vi "Teleop.vi"(10 "Match Info":T1={"Autonomous Elapsed Seconds"=0.0, "TeleOp Elapsed Seconds"=0.0, "Disabled Elapsed Seconds"=0.0, "Visited Autonomous"=FALSE, "Visited TeleOp"=FALSE, "Visited Disabled"=FALSE, "Autonomous Settings"={"Autonomous Style"=enum."Independent", "VI Refnum"=refnum}}, 11 "Call Context":T2) -> ()   [LabVIEW 2016]
doc: "This VI is called for each TeleOp packet received from the DS where the robot is not disabled. It is often used to read from the joysticks and update I/O or to update setpoints for timed control loops. It should complete and return within 20 milliseconds or it may miss DS packets."
uses:
  <vilib>/Rock Robotics/WPI/DriverStation/WPI_DriverStationDerivedRobotMode.ctl
  <vilib>/Rock Robotics/WPI/DriverStation/WPI_DriverStationMatch Info.ctl
  <vilib>/Rock Robotics/WPI/ThirdParty/CanMotor/TalonSRX/WPI_CANTalonSRX_APIFeedbackSelect.ctl
  <vilib>/Rock Robotics/WPI/ThirdParty/CanMotor/TalonSRX/WPI_CANTalonSRX_APIControlMode.ctl
  <vilib>/Rock Robotics/WPI/Utilities/WPI_GetSetVariantRefNum.vi
  <vilib>/Rock Robotics/Network Tables/NT Write Boolean Array.vi
  <vilib>/Rock Robotics/Network Tables/NT Write Numeric Array.vi
  <vilib>/Rock Robotics/Network Tables/NT Read Boolean.vi
  <vilib>/Rock Robotics/Network Tables/NT Read Number.vi
  Robot Global Data.vi
panel:
  out "Battery Voltage":dbl
  out "Current":dbl
  out "SensorPosRotations":dbl
  out "Motor output Plot":cluster{"Applied Throttle":dbl}(graph)
  out "Target RPM":dbl
  out "SensorRPM Velocity RPM":dbl
  out "Applied Output":dbl
  out "Speed Closed Loop Plots":cluster{dbl, "Sensor Velocity":dbl}(graph)
  in  "Enable":bool=TRUE
  in  "Reset":bool
  out "Table":string[][](table)
  out "Encoder Velocity":dbl
  out "Sample Slider 0":dbl(slide) scale=0.0..5.0
  out "Sample Boolean 1":bool
  out "Sample Boolean 0":bool
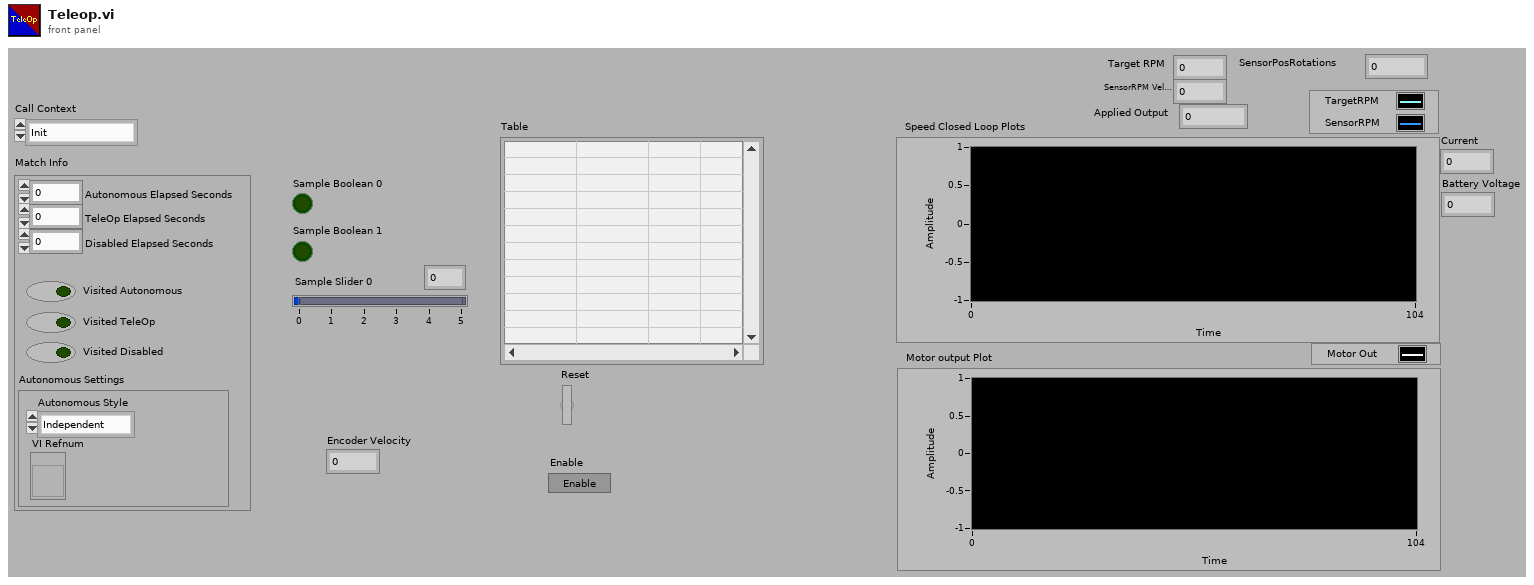
[diagram p1: front panel]
types:
  T1 = typedef "WPI_DriverStationMatch Info.ctl" = cluster{"Autonomous Elapsed Seconds":dbl, "TeleOp Elapsed Seconds":dbl, "Disabled Elapsed Seconds":dbl, "Visited Autonomous":bool, "Visited TeleOp":bool, "Visited Disabled":bool, "Autonomous Settings":cluster{"Autonomous Style":enum16{"Iterative", "Independent"}, "VI Refnum":refnum<vi>}}
  T2 = typedef "WPI_DriverStationDerivedRobotMode.ctl" = enum16{"Init", "Execute", "Stop"}
  T3 = typedef "WPI_CANTalonSRX_APIFeedbackSelect.ctl" = enum16{"Digital Quadrature Encoder", "Analog Potentiometer", "Analog Encoder", "Count on Quad-A (Rising-Edge)", "Count on Quad-A (Falling-Edge)", "CTR Magnetic Enc (Absolute)", "CTR Magnetic Enc (Relative)", "Pulse Width"}
  T4 = typedef "WPI_JoystickDevRef.ctl" = cluster{"Device":T5}
  T5 = typedef "WPI_JoystickDeviceEnum.ctl" = enum16{"USB 0", "USB 1", "USB 2", "USB 3", "USB 4", "USB 5"}
  T6 = typedef "WPI_MotorControlDeviceRef.ctl" = cluster{"DeviceStatus":errorcluster, "Type":T7, "PWM":cluster{"PWM Channel":T8, "DeadBand":T9}, "CAN":cluster{"Device Number":u8, "SetOutput VI Ref":variant, "GetOutput VI Ref":variant, "Enable VI Ref":variant, "Disable VI Ref":variant, "Data":variant}, "Invert":bool}
  T7 = typedef "WPI_MotorControlType.ctl" = enum16{"PWM", "CAN"}
  T8 = typedef "FPGA_DIOPWMChannel.ctl" = enum8{"PWM 0", "PWM 1", "PWM 2", "PWM 3", "PWM 4", "PWM 5", "PWM 6", "PWM 7", "PWM 8", "PWM 9", "PWM MXP 0", "PWM MXP 1", "PWM MXP 2", "PWM MXP 3", "PWM MXP 4", "PWM MXP 5", "PWM MXP 6", "PWM MXP 7", "PWM MXP 8", "PWM MXP 9", "Invalid"}
  T9 = typedef "WPI_PWMDeadband.ctl" = cluster{"Name":string, "maxPositivePwm":i32, "minPositivePwm":i32, "centerPwm":i32, "maxNegativePwm":i32, "minNegativePwm":i32, "angularRange":u16}
  T10 = typedef "WPI_RobotDriveDevRef.ctl" = cluster{"DevStatus":errorcluster, "Motors[]":T6[], "Square Inputs":bool, "Max Output":dbl}
  T11 = typedef "WPI_CANTalonSRX_GlobalStatus.ctl" = cluster{"Applied Throttle":dbl, "Module Enabled":bool, "CAN Error":errorcluster, "Closed Loop Error":dbl, "Forward Limit Switch Closed":bool, "Reverse Limit Switch Closed":bool, "Sensor Position":dbl, "Sensor Velocity":dbl, "Current":dbl, "Sticky Fault - Over Temp":bool, "Sticky Fault - Under Voltage":bool, "Sticky Fault - Forward Limit":bool, "Sticky Fault - Reverse Limit":bool, "Sticky Fault - Forward Soft Limit":bool, "Sticky Fault - Reverse Soft Limit":bool, "Brake is Enabled":bool, "Encoder Position":dbl, "Encoder Velocity":dbl, "Encoder Index Count":dbl, "Encoder A Pin State":bool, "Encoder B Pin State":bool, "Encoder Index Pin State":bool, "Analog In":dbl, "Analog In Velocity":dbl, "Temperature (C)":dbl, "Battery Voltage":dbl, "Control 5 Is Supported":bool, "Current Profile Slot Select":dbl, "Pos Div 8":bool, "Vel Div 4":bool, "Pulse Width Position":i32, "Pulse Width Velocity":i32, "Pulse Width Rise To Rise (us)":i32, "Pulse Width Rise To Fall (us)":i32, "Mot Prof Active Is Under Run":bool, "Mot Prof Active Has Under Run":bool, "Mot Prof Active Is Last":bool, "Mot Prof Active Velocity Only":bool, "Mot Prof Active Is Valid":bool, "Mot Prof Buffer Is Full":bool, "Mot Prof Active Profile Slot Select":i32, "Mot Prof NextID":i32, "Mot Prof Count":i32, "Mot Prof Active Velocity":dbl, "Mot Prof Active Position":dbl, "Mot Prof Output Enable":i32, "UsageFrame":u32}
  T12 = typedef "WPI_DigitalInputDevRef.ctl" = cluster{"DevStatus":errorcluster, "DIO Channel":T13}
  T13 = typedef "FPGA_DIOChannel.ctl" = enum8{"DIO 0", "DIO 1", "DIO 2", "DIO 3", "DIO 4", "DIO 5", "DIO 6", "DIO 7", "DIO 8", "DIO 9", "DIO MXP 0", "DIO MXP 1", "DIO MXP 2", "DIO MXP 3", "DIO MXP 4", "DIO MXP 5", "DIO MXP 6", "DIO MXP 7", "DIO MXP 8", "DIO MXP 9", "DIO MXP 10", "DIO MXP 11", "DIO MXP 12", "DIO MXP 13", "DIO MXP 14", "DIO MXP 15", "SPI Port CS1", "SPI Port CS2", "SPI Port CS3", "SPI Port MISO", "SPI Port MOSI", "Invalid"}
  T14 = typedef "WPI_CANTalonSRX_APIControlMode.ctl" = enum8{"Percent VBus", "Speed", "Position", "Slave", "Unchanged / Invalid", "Voltage Compensation", "Current", "Motion Profile", "Motion Magic"}
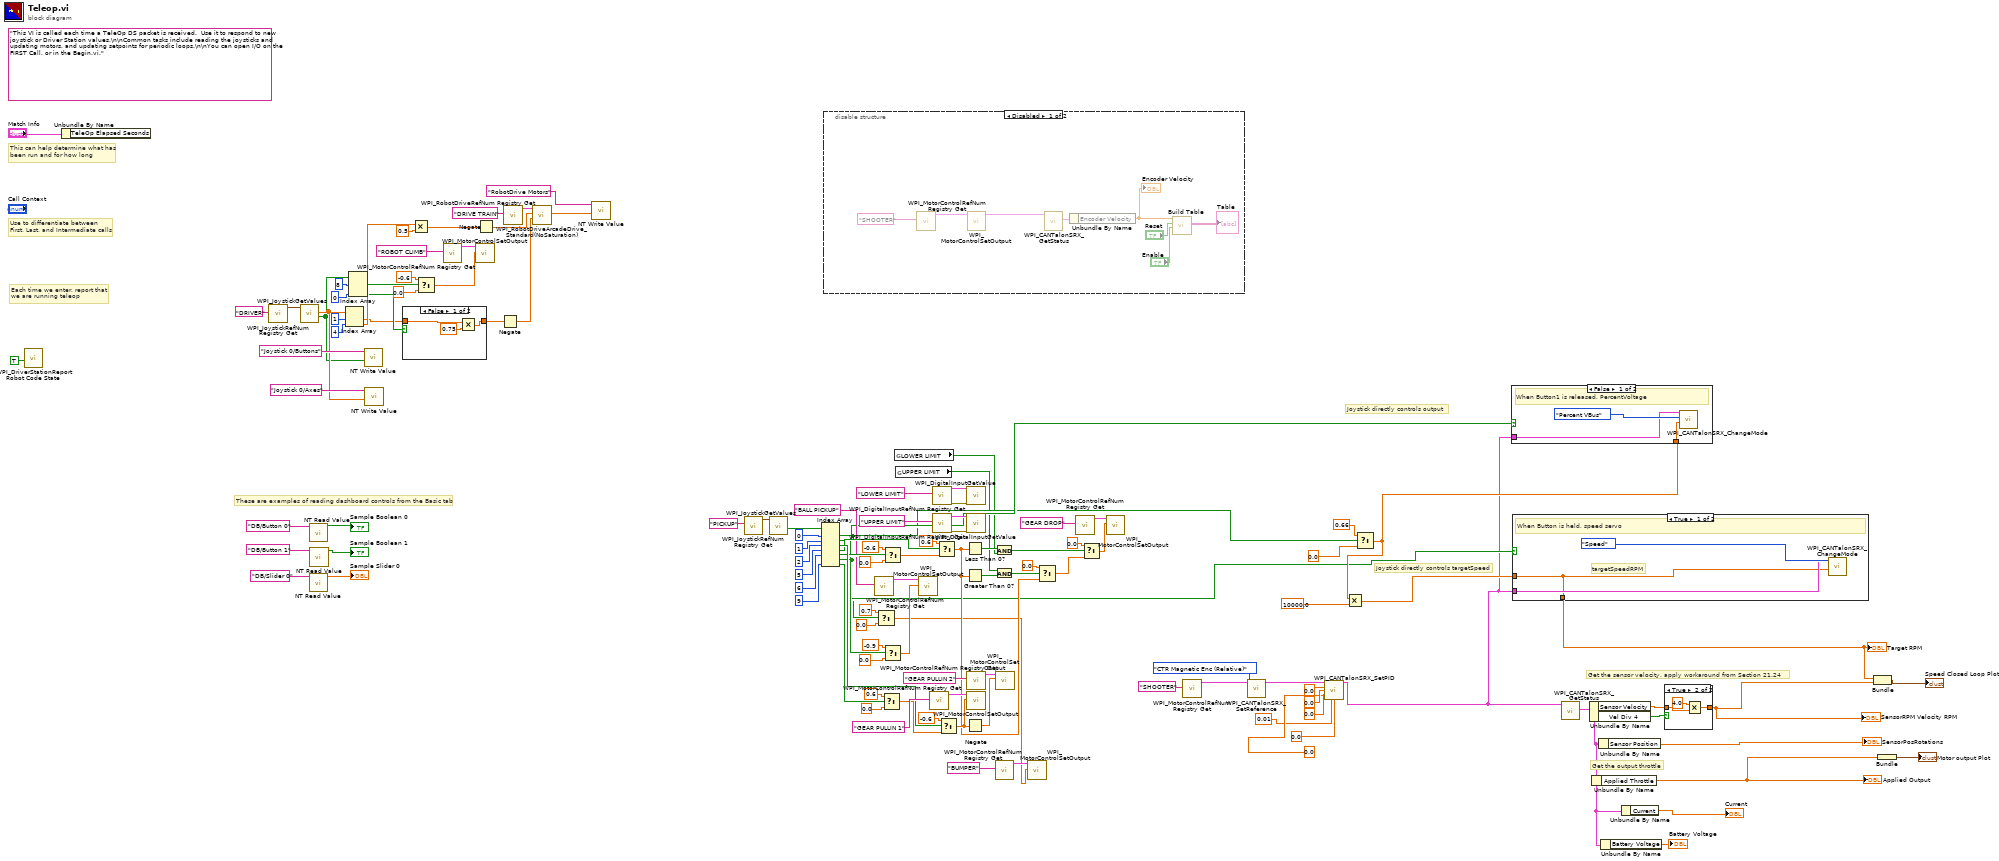
[diagram p0: block diagram]
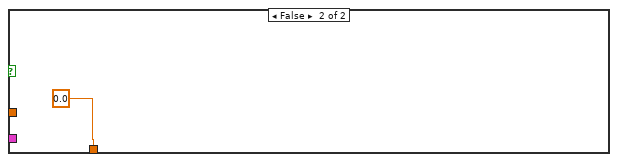
[diagram p6: hidden frame]
diagram:
  (unwired) "This VI is called each time a TeleOp DS packet is received.  Use it to respond to new joystick or Driver Station values.\n\nCommon tasks include reading the joysticks and updating motors, and updating setpoints for periodic loops.\n\nYou can open I/O on the FIRST Call, or in the Begin.vi."
  # "Get the output throttle"
  # "Get the sensor velocity, apply workaround from Section 21.24"
  # "Joystick directly controls targetSpeed"
  # "Joystick directly controls output"
  # "These are examples of reading dashboard controls from the Basic tab"
  # "Each time we enter, report that\nwe are running teleop"
  # "Use to differentiate between\nFirst, Last, and Intermediate calls"
  # "This can help determine what has\nbeen run and for how long"
  n1 = call <vilib>:"WPI_DriverStationReport Robot Code State.vi"("TeleOp"=TRUE ("Autonomous")) -> ()  [unwired: 10 in, 1 out]
  n2 = Unbundle By Name("Match Info") -> ()  [unwired: 1 out]
  n3 = call <vilib>:"WPI_JoystickRefNum Registry Get.vi"("refnum name"="DRIVER") -> ("JoystickDevRef"=w118:T4)  [unwired: 1 in, 9 out]
  n4 = call <vilib>:"WPI_JoystickGetValues.vi"("JoystickDevRef"=w118) -> ("Buttons"=w76:bool[], "Axes"=w114:dbl[])  [unwired: 6 in, 3 out]
  n5 = call-poly <vilib>:"NT Read Value.vi"("Name"="DB/Button 0" ("refnum name")) -> ("Boolean"=→"Sample Boolean 0":bool)  [unwired: 9 in, 1 out]
  n6 = call-poly <vilib>:"NT Read Value.vi"("Name"="DB/Slider 0" ("refnum name")) -> ("Numeric"=→"Sample Slider 0":dbl)  [unwired: 9 in, 1 out]
  n7 = call-poly <vilib>:"NT Read Value.vi"("Name"="DB/Button 1" ("refnum name")) -> ("Boolean"=→"Sample Boolean 1":bool)  [unwired: 9 in, 1 out]
  n8 = Index Array(array=w114, index #1=1 ("index"), index #2=4 ("index")) -> (element #1=w13:dbl, element #2=w66:dbl)
  n9 = Index Array(array=w76, index #1=8 ("index"), index #3=0 ("index")) -> (element #1=w72:bool, element #3=w14:bool)  [unwired: 1 in, 1 out]
  n10 = call-poly <vilib>:"NT Write Value.vi"("Boolean Array"=w76, "Name"="Joystick 0/Buttons") -> ()  [unwired: 9 in, 1 out]
  n11 = call-poly <vilib>:"NT Write Value.vi"("Numeric Array"=w114, "Name"="Joystick 0/Axes") -> ()  [unwired: 9 in, 1 out]
  n12 = case shown="False" w14 {
    tunnel: [w124 w126] -> w12
    tunnel: w13 -> [w123 w126]
    frame False {
      n13 = Multiply(x=w123, y=0.75) -> (x*y=w124:dbl)
    }
    frame True {
    }
  }
  n14 = Multiply(x=w66, y=0.5) -> (x*y=w57:dbl)
  n15 = Select(t=-0.6, s=w72, f=0.0) -> (s? t:f=w73:dbl)
  n16 = call <vilib>:"WPI_MotorControlRefNum Registry Get.vi"("refnum name"="ROBOT CLIMB") -> ("MotorControlDevRef"=w74:T6)  [unwired: 9 in, 1 out]
  n17 = call <vilib>:"WPI_MotorControlSetOutput.vi"("Output"=w73, "MotorControlDevRef"=w74) -> ()  [unwired: 7 in, 3 out]
  n18 = Negate(x=w57) -> (-x=w56:dbl)
  n19 = Negate(x=w12) -> (-x=w58:dbl)
  n20 = call <vilib>:"WPI_RobotDriveRefNum Registry Get.vi"("refnum name"="DRIVE TRAIN") -> ("RobotDriveDevRef"=w120:T10)  [unwired: 1 in, 9 out]
  n21 = call <vilib>:"WPI_RobotDriveArcadeDrive_Standard(NoSaturation).vi"("Y axis value"=w58, "X axis value"=w56, "RobotDriveDevRef"=w120) -> ("Motor Values"=w107:dbl[])  [unwired: 1 in, 7 out]
  n22 = call-poly <vilib>:"NT Write Value.vi"("Numeric Array"=w107, "Name"="RobotDrive Motors") -> ()  [unwired: 9 in, 1 out]
  n23 = call <vilib>:"WPI_JoystickRefNum Registry Get.vi"("refnum name"="PICKUP") -> ("JoystickDevRef"=w105:T4)  [unwired: 1 in, 9 out]
  n24 = call <vilib>:"WPI_JoystickGetValues.vi"("JoystickDevRef"=w105) -> ("Buttons"=w103:bool[])  [unwired: 6 in, 4 out]
  n25 = Index Array(array=w103, index #1=0 ("index"), index #2=1 ("index"), index #3=2 ("index"), index #4=5 ("index"), index #5=6 ("index"), index #7=9 ("index")) -> (element #1=w22:bool, element #2=w79:bool, element #3=w86:bool, element #4=w85:bool, element #5=w84:bool, element #6=w25:bool, element #7=w8:bool)  [unwired: 1 in]
  n26 = disable-structure shown="Disabled" {
    frame Disabled {
      n27 = call <vilib>:"WPI_MotorControlRefNum Registry Get.vi"("refnum name"="SHOOTER") -> ("MotorControlDevRef"=w127:T6)  [unwired: 9 in, 1 out]
      n28 = call <vilib>:"WPI_MotorControlSetOutput.vi"("MotorControlDevRef"=w127) -> ("MotorControlDevRef"=w134:T6)  [unwired: 8 in, 2 out]
      n29 = call <vilib>:"WPI_CANTalonSRX_GetStatus.vi"("CAN Talon SRX Ref"=w134) -> ("Talon SRX Status"=w133:T11)  [unwired: 8 in, 2 out]
      n30 = Unbundle By Name(w133) -> ("Encoder Velocity"=w131:dbl)
      "Encoder Velocity" <- w131
      n31 = call "Build Table"("Enable"="Enable", "Reset"="Reset", "Signals"=w131) -> ("Table"=→"Table":string[][])  [unwired: 2 in, 6 out]
    }
    frame Enabled {
    }
  }
  n32 = call <vilib>:"WPI_MotorControlRefNum Registry Get.vi"("refnum name"="BALL PICKUP") -> ("MotorControlDevRef"=w83:T6)  [unwired: 9 in, 1 out]
  n33 = Select(t=0.7, s=w22, f=0.0) -> (s? t:f=w19:dbl)
  n34 = Select(t=0.6, s=w8, f=0.0) -> (s? t:f=w10:dbl)
  n35 = Select(t=-0.6, s=w84, f=0.0) -> (s? t:f=w54:dbl)
  n36 = Select(t=-0.9, s=w79, f=0.0) -> (s? t:f=w81:dbl)
  n37 = global read "Robot Global Data.vi" "LOWER LIMIT"() -> (w2:bool)
  n38 = global read "Robot Global Data.vi" "UPPER LIMIT"() -> (w1:bool)
  n39 = call <vilib>:"WPI_MotorControlSetOutput.vi"("Output"=w81, "MotorControlDevRef"=w83) -> ()  [unwired: 7 in, 3 out]
  n40 = call <vilib>:"WPI_MotorControlRefNum Registry Get.vi"("refnum name"="GEAR PULLIN 1") -> ("MotorControlDevRef"=w101:T6)  [unwired: 9 in, 1 out]
  n41 = call <vilib>:"WPI_DigitalInputRefNum Registry Get.vi"("refnum name"="LOWER LIMIT") -> ("error out"=w61:errorcluster, "DigitalInputDevRef"=w62:T12)  [unwired: 9 in]
  n42 = call <vilib>:"WPI_DigitalInputRefNum Registry Get.vi"("refnum name"="UPPER LIMIT") -> ("error out"=w64:errorcluster, "DigitalInputDevRef"=w63:T12)  [unwired: 9 in]
  n43 = Select(t=0.6, s=w85, f=w54) -> (s? t:f=w48:dbl)
  n44 = Select(t=-0.6, s=w86, f=w10) -> (s? t:f=w96:dbl)
  n45 = Less Than 0?(x=w48) -> (x < 0?=w50:bool)
  n46 = Greater Than 0?(x=w48) -> (x > 0?=w51:bool)
  n47 = Negate(x=w96) -> (-x=w95:dbl)
  n48 = call <vilib>:"WPI_DigitalInputGetValue.vi"("error in (no error)"=w61, "DigitalInputDevRef"=w62) -> ()  [unwired: 7 in, 3 out]
  n49 = call <vilib>:"WPI_DigitalInputGetValue.vi"("error in (no error)"=w64, "DigitalInputDevRef"=w63) -> ()  [unwired: 7 in, 3 out]
  n50 = call <vilib>:"WPI_MotorControlRefNum Registry Get.vi"("refnum name"="GEAR PULLIN 2") -> ("MotorControlDevRef"=w98:T6)  [unwired: 9 in, 1 out]
  n51 = call <vilib>:"WPI_MotorControlSetOutput.vi"("Output"=w96, "MotorControlDevRef"=w101) -> ()  [unwired: 7 in, 3 out]
  n52 = And(x=w50, y=w2) -> (x .and. y?=w52:bool)
  n53 = And(x=w1, y=w51) -> (x .and. y?=w53:bool)
  n54 = call <vilib>:"WPI_MotorControlRefNum Registry Get.vi"("refnum name"="BUMPER") -> ("MotorControlDevRef"=w24:T6)  [unwired: 9 in, 1 out]
  n55 = call <vilib>:"WPI_MotorControlSetOutput.vi"("Output"=w95, "MotorControlDevRef"=w98) -> ()  [unwired: 7 in, 3 out]
  n56 = call <vilib>:"WPI_MotorControlSetOutput.vi"("Output"=w19, "MotorControlDevRef"=w24) -> ()  [unwired: 7 in, 3 out]
  n57 = Select(t=0.0, s=w53, f=w48) -> (s? t:f=w46:dbl)
  n58 = call <vilib>:"WPI_MotorControlRefNum Registry Get.vi"("refnum name"="GEAR DROP") -> ("MotorControlDevRef"=w93:T6)  [unwired: 9 in, 1 out]
  n59 = Select(t=0.0, s=w52, f=w46) -> (s? t:f=w55:dbl)
  n60 = call <vilib>:"WPI_MotorControlSetOutput.vi"("Output"=w55, "MotorControlDevRef"=w93) -> ()  [unwired: 7 in, 3 out]
  n61 = call <vilib>:"WPI_MotorControlRefNum Registry Get.vi"("refnum name"="SHOOTER") -> ("MotorControlDevRef"=w36:T6)  [unwired: 9 in, 1 out]
  n62 = call <vilib>:"WPI_CANTalonSRX_SetReference.vi"("Feedback Reference"=WPI_CANTalonSRX_APIFeedbackSelect."CTR Magnetic Enc (Relative)", "CAN Talon SRX Ref"=w36) -> ("CAN Talon SRX Ref"=w35:T6)  [unwired: 8 in, 1 out]
  n63 = call <vilib>:"WPI_CANTalonSRX_SetPID.vi"("CAN Talon SRX Ref"=w35, "P"=0.0, "I"=0.0, "D"=0.0, "F"=0.01, "I Zone"=0.0, "Ramp Rate"=0.0) -> ("CAN Talon SRX Ref"=w6:T6)  [unwired: 7 in, 1 out]
  n64 = Select(t=0.66 ("Output"), s=w22, f=0.0) -> (s? t:f=w27:dbl)
  n65 = Multiply(x=w27, y=10000.0) -> (x*y=w30:dbl)
  n66 = case shown="False" w25 {
    tunnel: w6 -> [w136 _]
    tunnel: w27 -> [w135 _]
    frame False {
      # "When Button1 is released, PercentVoltage"
      n67 = call <vilib>:"WPI_CANTalonSRX_ChangeMode.vi"("Output"=w135, "Control Mode"=WPI_CANTalonSRX_APIControlMode."Percent VBus", "CAN Talon SRX Ref"=w136) -> ()  [unwired: 7 in, 2 out]
    }
    frame True {
    }
  }
  n68 = case shown="True" w25 {
    tunnel: w30 -> [w138 _]
    tunnel: w6 -> [w139 _]
    tunnel: [w138 0.0 ("x")] -> w29
    frame True {
      # "targetSpeedRPM"
      # "When Button is held, speed servo"
      n69 = call <vilib>:"WPI_CANTalonSRX_ChangeMode.vi"("Output"=w138, "Control Mode"=WPI_CANTalonSRX_APIControlMode."Speed", "CAN Talon SRX Ref"=w139) -> ()  [unwired: 7 in, 2 out]
    }
    frame False {
    }
  }
  "Target RPM" <- w29
  n70 = call <vilib>:"WPI_CANTalonSRX_GetStatus.vi"("CAN Talon SRX Ref"=w6) -> ("Talon SRX Status"=w17:T11)  [unwired: 8 in, 2 out]
  n71 = Unbundle By Name(w17) -> ("Sensor Velocity"=w39:dbl, "Vel Div 4"=w38:bool)
  n72 = Unbundle By Name(w17) -> ("Applied Throttle"=w31:dbl)
  "Applied Output" <- w31
  n73 = Unbundle By Name(w17) -> ("Sensor Position"=→"SensorPosRotations":dbl)
  n74 = Unbundle By Name(w17) -> ("Battery Voltage"=→"Battery Voltage":dbl)
  n75 = Unbundle By Name(w17) -> ("Current"=→"Current":dbl)
  n76 = case shown="True" w38 {
    tunnel: [w142 w144] -> w37
    tunnel: w39 -> [w142 w143]
    frame False {
    }
    frame True {
      n77 = Multiply(x=4.0, y=w143) -> (x*y=w144:dbl)
    }
  }
  "SensorRPM Velocity RPM" <- w37
  n78 = Bundle("x"=w29, "Sensor Velocity"=w37) -> (→"Speed Closed Loop Plots":cluster{"x":dbl, "Sensor Velocity":dbl})  [unwired: 1 in]
  n79 = Bundle("Applied Throttle"=w31) -> (→"Motor output Plot":cluster{"Applied Throttle":dbl})  [unwired: 1 in]
